vi "iTCread.vi"(0 "VISA resource name":refnum<visa-resource-name>, 1 "iTCreadCtrl":T1, 3 "error in (no error)":errorcluster) -> (7 "VISA resource name out":refnum<visa-resource-name>, 8 "number":dbl, 9 "read buffer":string, 10 "error out":errorcluster)   [LabVIEW 2017]
uses:
  controls/iTCreadCtrl.ctl
  <vilib>/regexp/Match Regular Expression.xnode
panel:
  out "read buffer 2":string
  out "after match":string
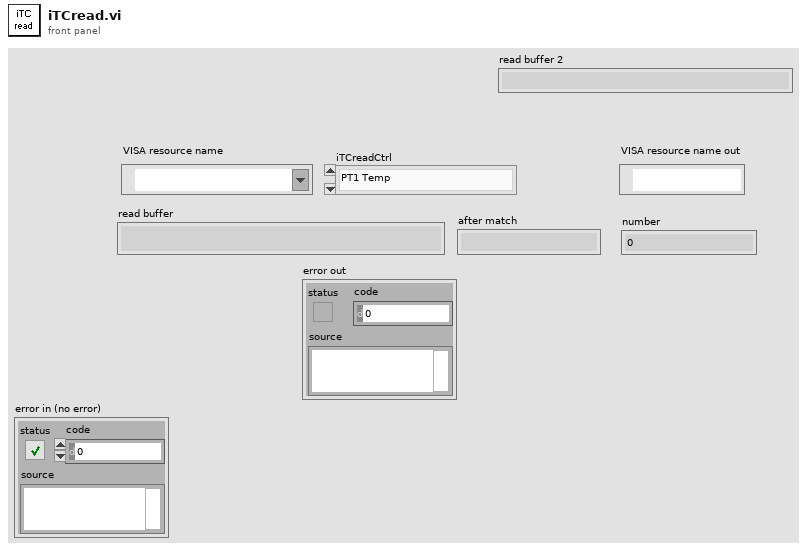
[diagram p1: front panel]
types:
  T1 = typedef "iTCreadCtrl.ctl" = enum16{"PT1 Temp", "PT2 Temp", "Sample Temp", "VTI Temp", "Needle Valve", "VTI Heater Power", "Sample Heater Power", "VTI Pressure"}
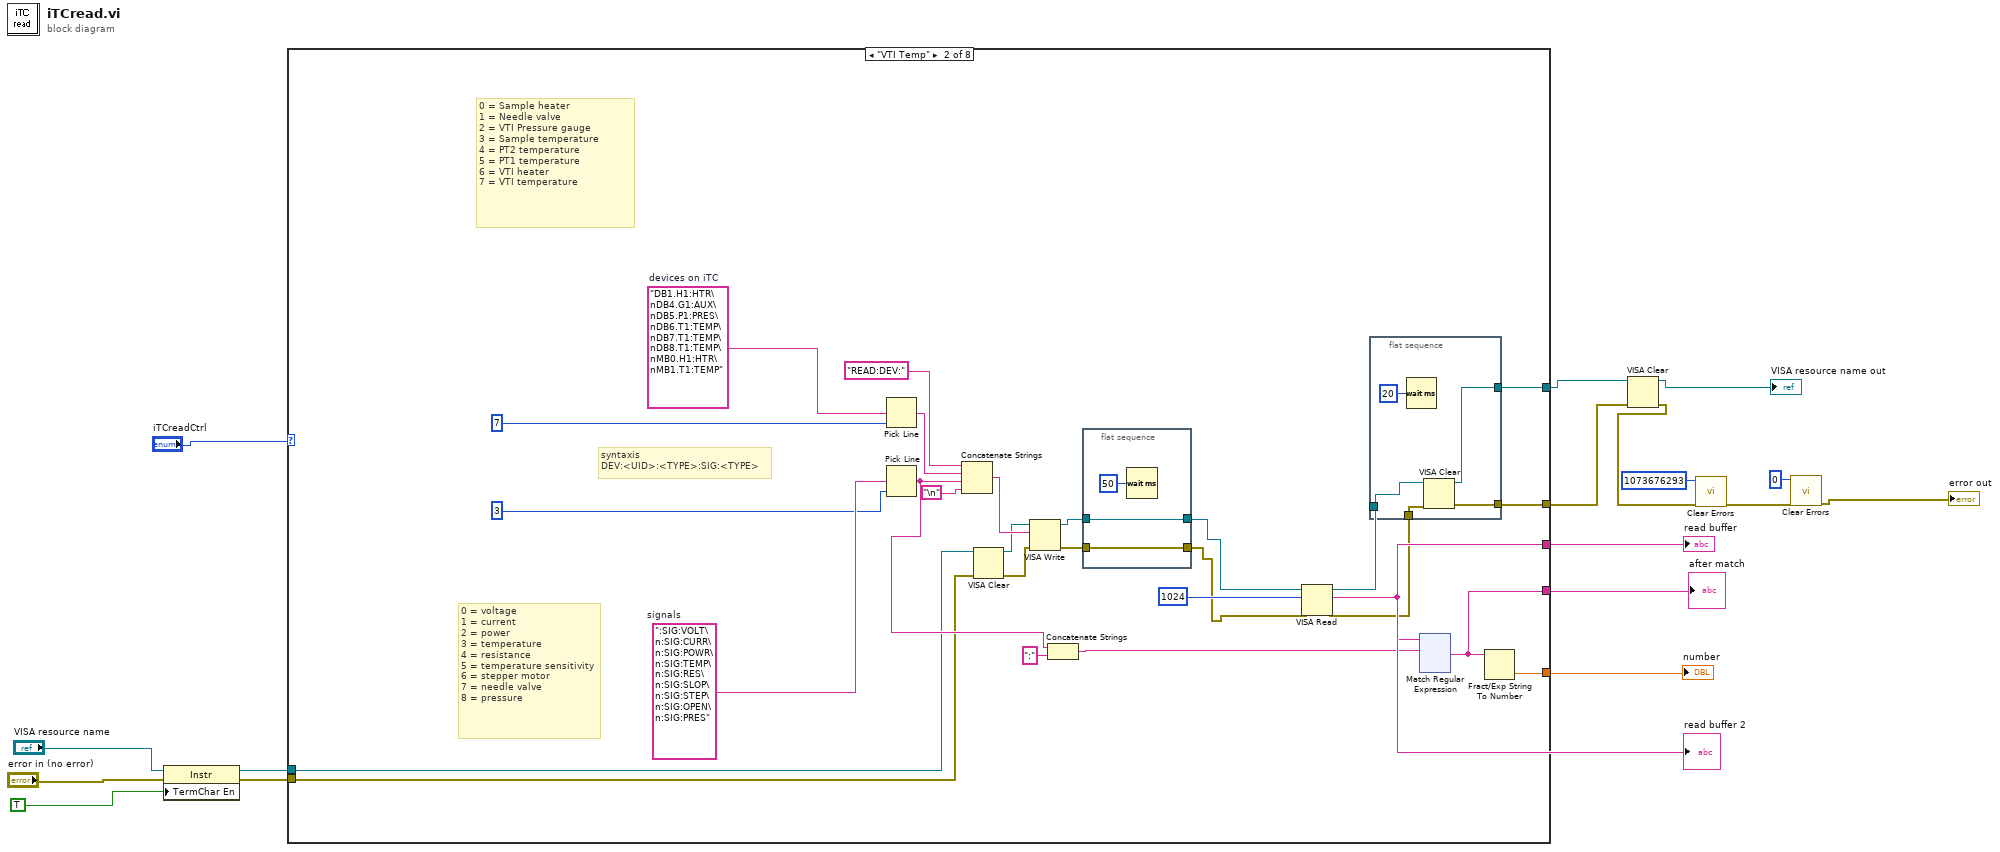
[diagram p0: block diagram]
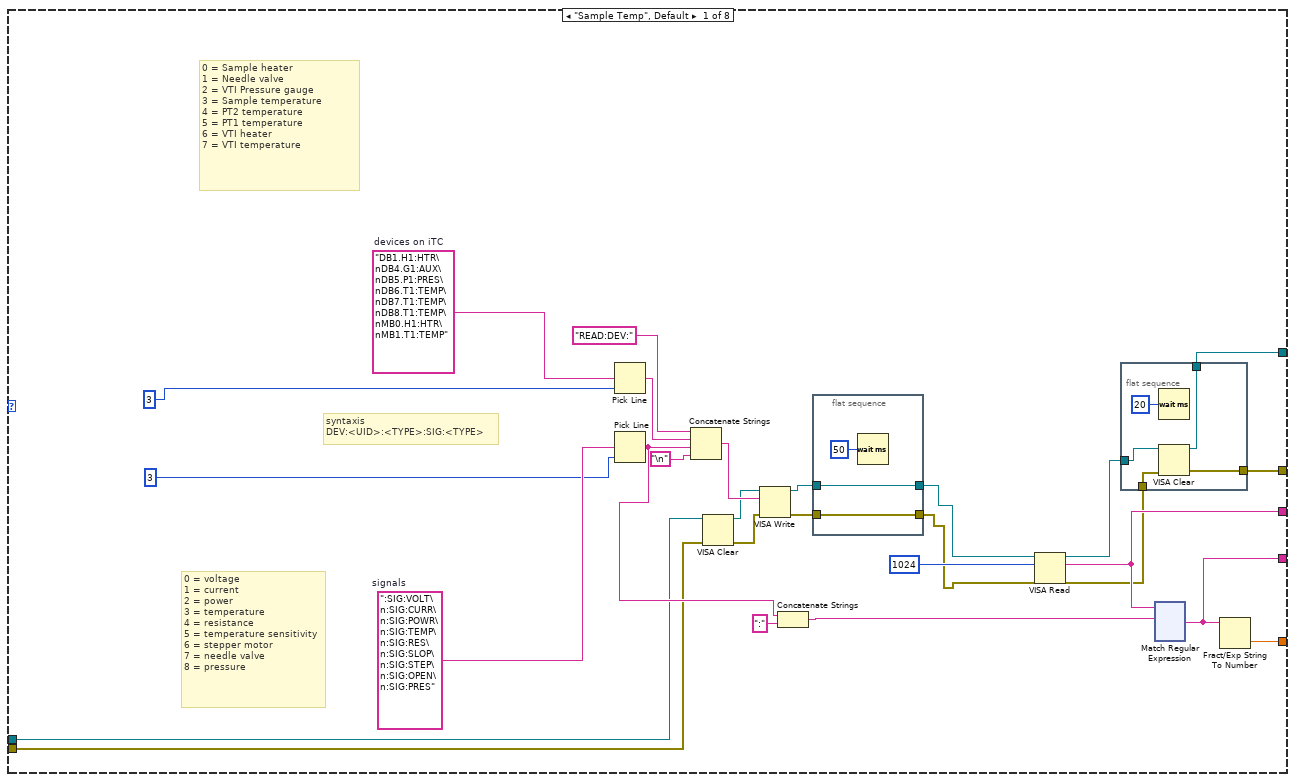
[diagram p2: hidden frame]
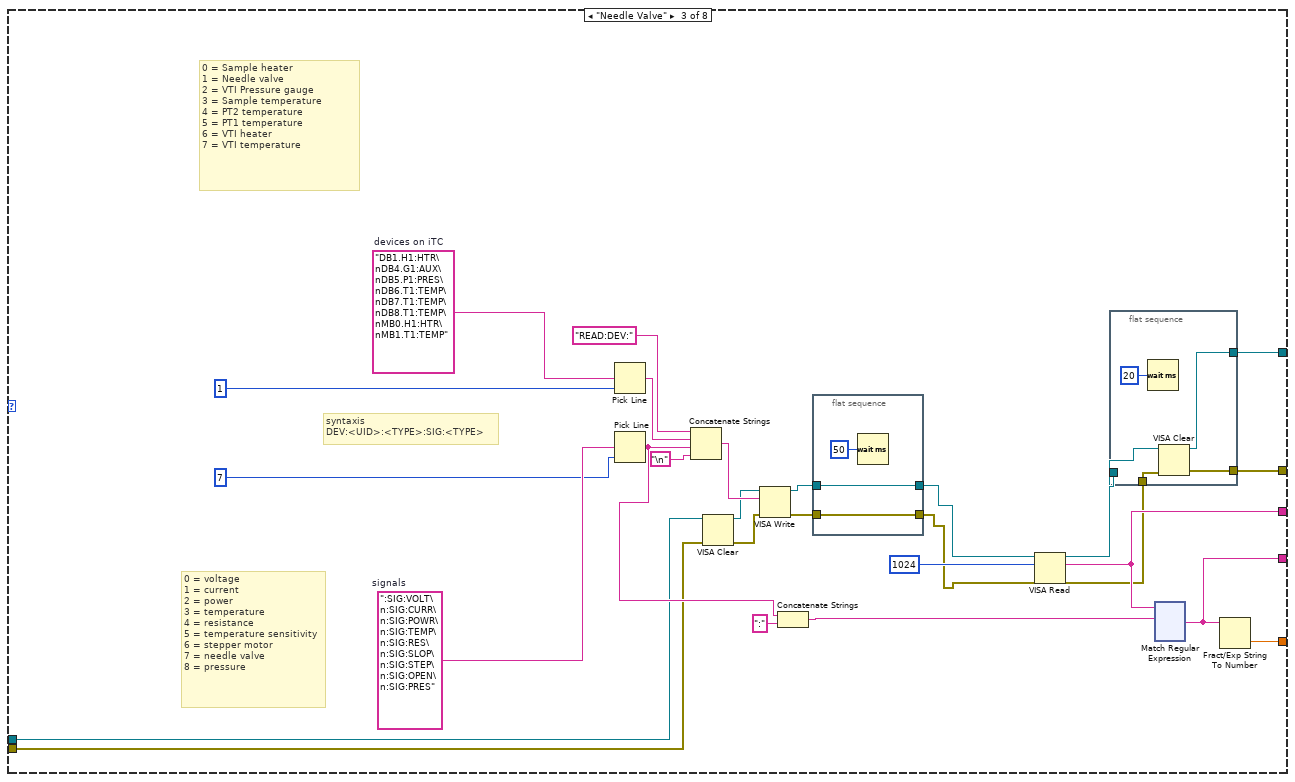
[diagram p3: hidden frame]
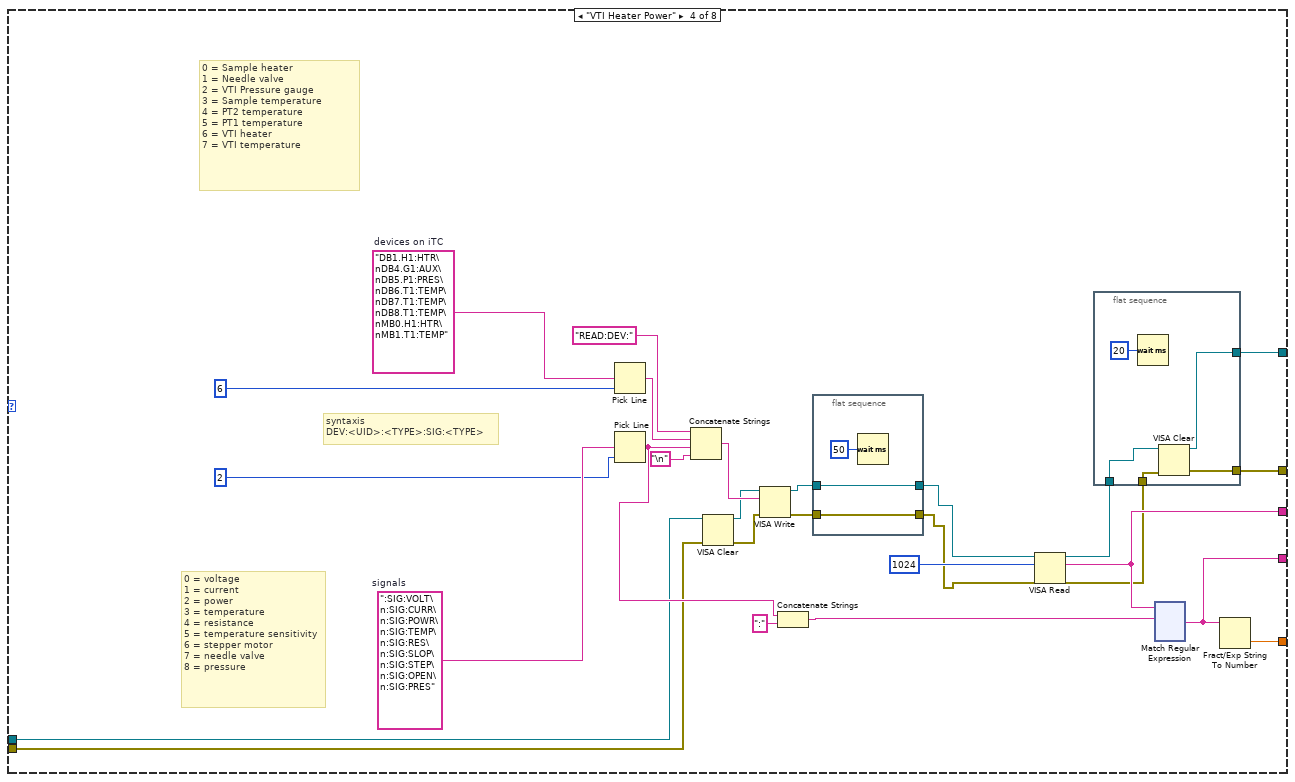
[diagram p4: hidden frame]
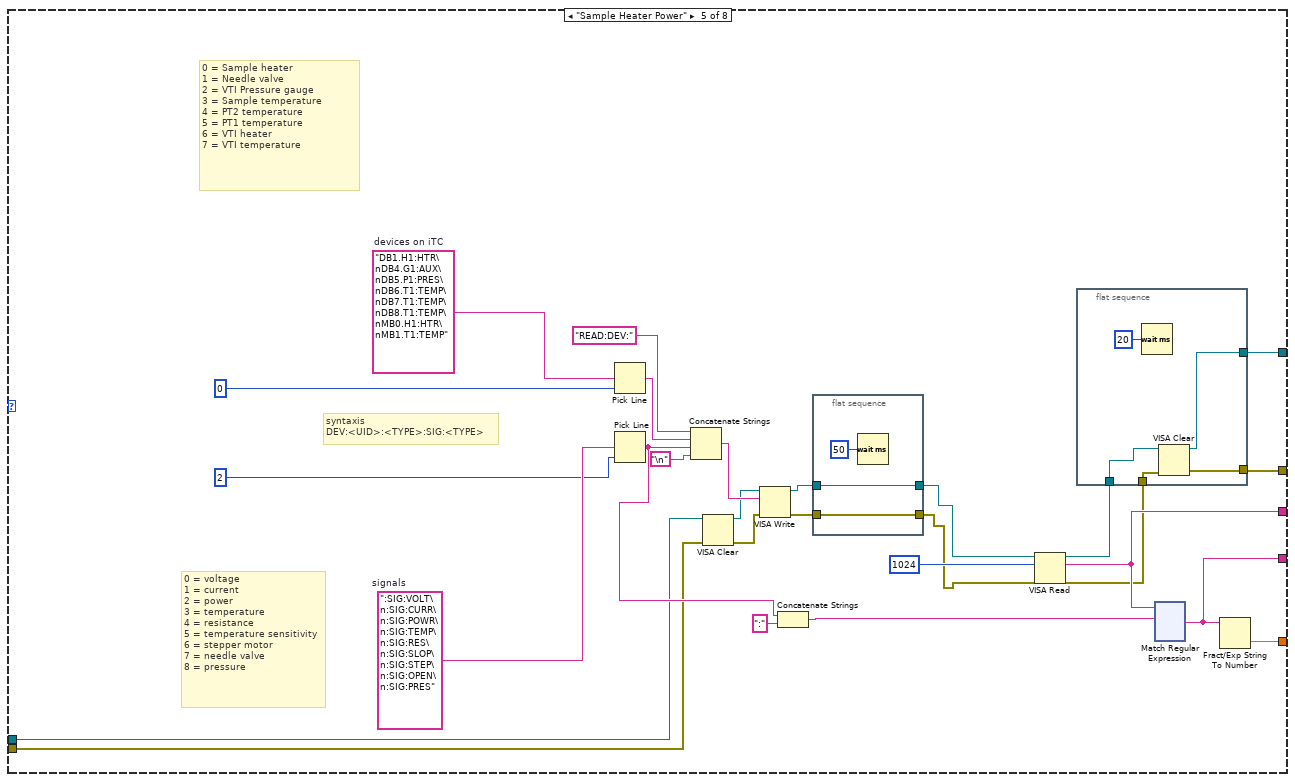
[diagram p5: hidden frame]
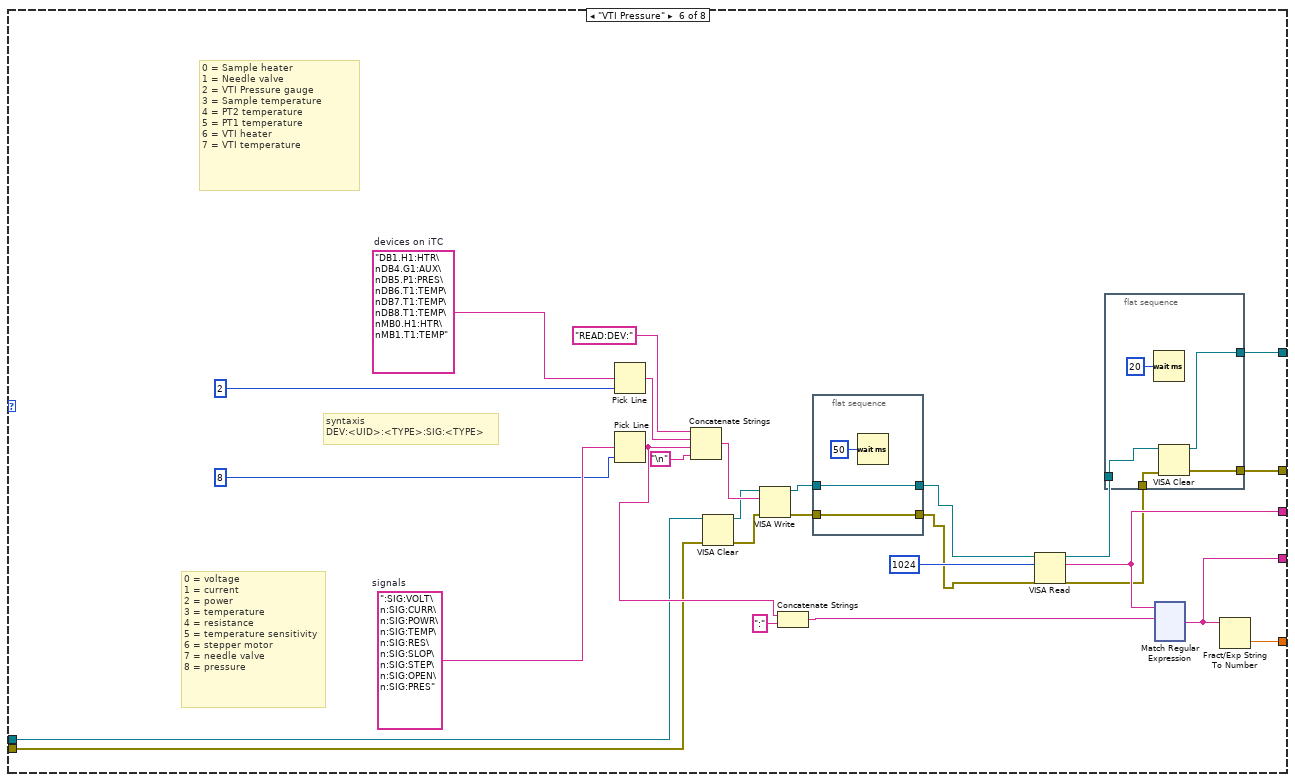
[diagram p6: hidden frame]
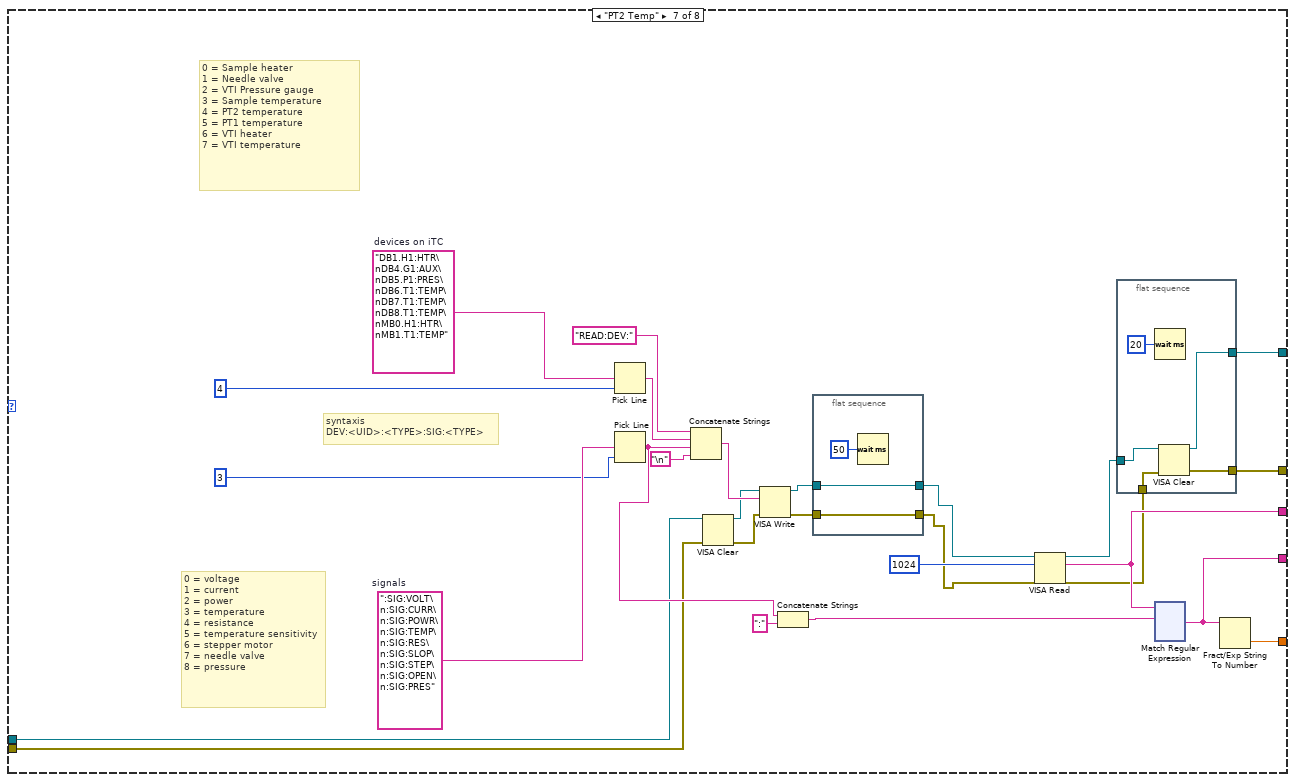
[diagram p7: hidden frame]
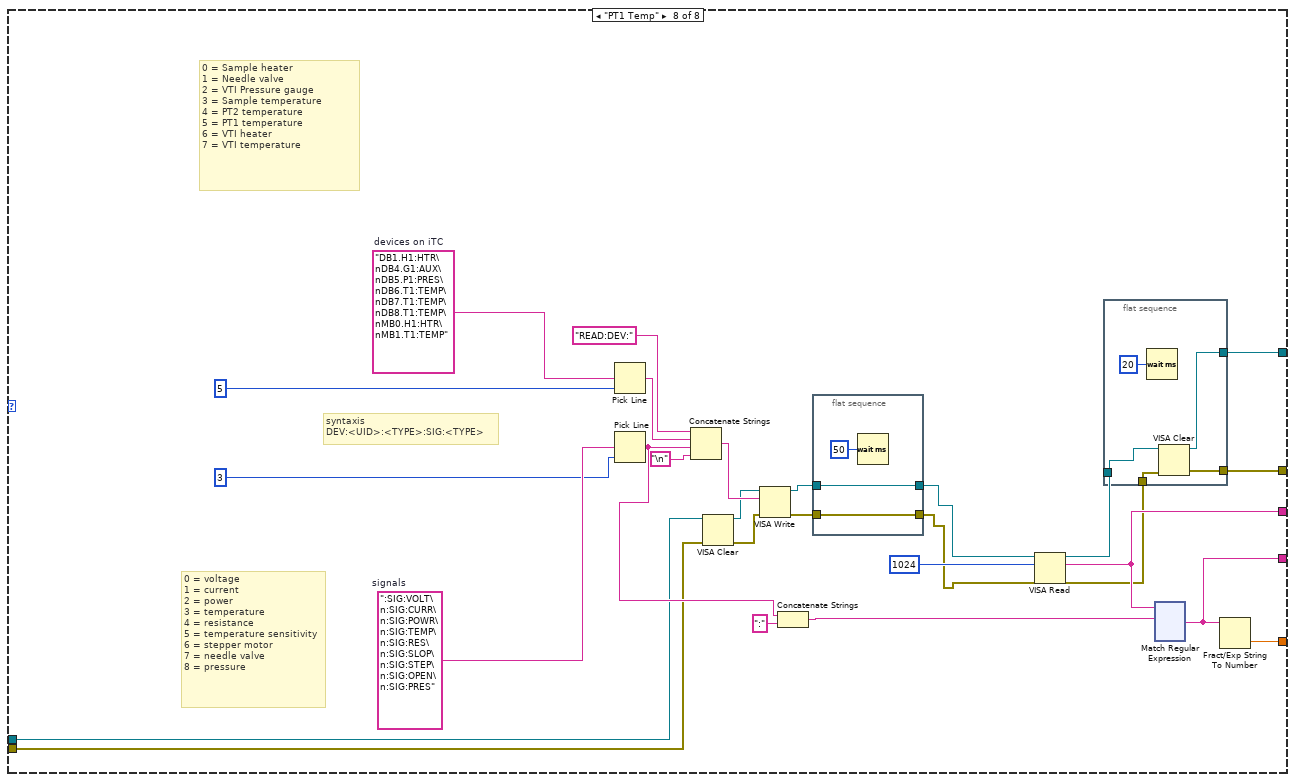
[diagram p8: hidden frame]
diagram:
  n1 = property class="Instr"(reference="VISA resource name", error in="error in (no error)", "TermChar En"=TRUE ("Message Based Settings:Termination Character Enable")) -> (reference out=w11:refnum<visa-resource-name>, error out=w12:errorcluster)
  n2 = case shown="\"VTI Temp\"" "iTCreadCtrl" {
    tunnel: [w44 w190 w336 w482 w628 w774 w920 w1066] -> w17
    tunnel: [w43 w189 w335 w481 w627 w773 w919 w1065] -> w16
    tunnel: [w42 w188 w334 w480 w626 w772 w918 w1064] -> w15
    tunnel: [w41 w187 w333 w479 w625 w771 w917 w1063] -> w2
    tunnel: [w40 w186 w332 w478 w624 w770 w916 w1062] -> w4
    tunnel: w12 -> [w23 w169 w315 w461 w607 w753 w899 w1045]
    tunnel: w11 -> [w22 w168 w314 w460 w606 w752 w898 w1044]
    frame "Sample Temp", Default {
      w36 = ":SIG:VOLT\n:SIG:CURR\n:SIG:POWR\n:SIG:TEMP\n:SIG:RES\n:SIG:SLOP\n:SIG:STEP\n:SIG:OPEN\n:SIG:PRES"  # signals
      w39 = "DB1.H1:HTR\nDB4.G1:AUX\nDB5.P1:PRES\nDB6.T1:TEMP\nDB7.T1:TEMP\nDB8.T1:TEMP\nMB0.H1:HTR\nMB1.T1:TEMP"  # devices on iTC
      # "0 = Sample heater\n1 = Needle valve\n2 = VTI Pressure gauge\n3 = Sample temperature\n4 = PT2 temperature\n5 = PT1 temperature\n6 = VTI heater\n7 = VTI temperature"
      # "0 = voltage\n1 = current\n2 = power\n3 = temperature\n4 = resistance\n5 = temperature sensitivity\n6 = stepper motor\n7 = needle valve\n8 = pressure"
      # "syntaxis\nDEV:<UID>:<TYPE>:SIG:<TYPE>"
      n3 = Pick Line(multi-line string=w39, line index=3) -> (output string=w37:string)  [unwired: 1 in]
      n4 = Pick Line(multi-line string=w36, line index=3) -> (output string=w33:string)  [unwired: 1 in]
      n5 = Concatenate Strings("READ:DEV:" ("write buffer"), w37, w33, "\n") -> (w35:string)
      n6 = VISA Clear(VISA resource name=w22, error in (no error)=w23) -> (VISA resource name out=w26:refnum<visa-resource-name>, error out=w27:errorcluster)
      n7 = VISA Write(VISA resource name=w26, write buffer=w35, error in (no error)=w27) -> (VISA resource name out=w21:refnum<visa-resource-name>, error out=w20:errorcluster)  [unwired: 1 out]
      n8 = Concatenate Strings(w33, ":" ("string")) -> (w32:string)
      n9 = flat-sequence {
        tunnel: w21 -> [w52]
        tunnel: w20 -> [w51]
        tunnel: [w52] -> w19
        tunnel: [w51] -> w18
        frame #0 {
          n10 = Wait (ms)(milliseconds to wait=u32 50) -> ()  [unwired: 1 out]
        }
      }
      n11 = VISA Read(VISA resource name=w19, byte count=u32 1024, error in (no error)=w18) -> (VISA resource name out=w25:refnum<visa-resource-name>, read buffer=w42:string, error out=w28:errorcluster)  [unwired: 1 out]
      n12 = flat-sequence {
        tunnel: [w49] -> w41
        tunnel: [w48] -> w40
        tunnel: w28 -> [w47]
        tunnel: w25 -> [w46]
        frame #0 {
          n13 = Wait (ms)(milliseconds to wait=u32 20) -> ()  [unwired: 1 out]
          n14 = VISA Clear(VISA resource name=w46, error in (no error)=w47) -> (VISA resource name out=w48:refnum<visa-resource-name>, error out=w49:errorcluster)
        }
      }
      n15 = xnode "Match Regular Expression"("input string"=w42, "regular expression"=w32) -> ("after match"=w44:string)  [unwired: 4 in, 4 out]
      n16 = Fract/Exp String To Number(string=w44) -> (number=w43:dbl)  [unwired: 3 in, 1 out]
    }
    frame "VTI Temp" {
      w182 = ":SIG:VOLT\n:SIG:CURR\n:SIG:POWR\n:SIG:TEMP\n:SIG:RES\n:SIG:SLOP\n:SIG:STEP\n:SIG:OPEN\n:SIG:PRES"  # signals
      w185 = "DB1.H1:HTR\nDB4.G1:AUX\nDB5.P1:PRES\nDB6.T1:TEMP\nDB7.T1:TEMP\nDB8.T1:TEMP\nMB0.H1:HTR\nMB1.T1:TEMP"  # devices on iTC
      # "0 = Sample heater\n1 = Needle valve\n2 = VTI Pressure gauge\n3 = Sample temperature\n4 = PT2 temperature\n5 = PT1 temperature\n6 = VTI heater\n7 = VTI temperature"
      # "0 = voltage\n1 = current\n2 = power\n3 = temperature\n4 = resistance\n5 = temperature sensitivity\n6 = stepper motor\n7 = needle valve\n8 = pressure"
      # "syntaxis\nDEV:<UID>:<TYPE>:SIG:<TYPE>"
      n17 = Pick Line(multi-line string=w185, line index=7) -> (output string=w183:string)  [unwired: 1 in]
      n18 = Pick Line(multi-line string=w182, line index=3) -> (output string=w179:string)  [unwired: 1 in]
      n19 = Concatenate Strings("READ:DEV:" ("write buffer"), w183, w179, "\n") -> (w181:string)
      n20 = VISA Clear(VISA resource name=w168, error in (no error)=w169) -> (VISA resource name out=w172:refnum<visa-resource-name>, error out=w173:errorcluster)
      n21 = VISA Write(VISA resource name=w172, write buffer=w181, error in (no error)=w173) -> (VISA resource name out=w167:refnum<visa-resource-name>, error out=w166:errorcluster)  [unwired: 1 out]
      n22 = Concatenate Strings(w179, ":" ("string")) -> (w178:string)
      n23 = flat-sequence {
        tunnel: w167 -> [w198]
        tunnel: w166 -> [w197]
        tunnel: [w198] -> w165
        tunnel: [w197] -> w164
        frame #0 {
          n24 = Wait (ms)(milliseconds to wait=u32 50) -> ()  [unwired: 1 out]
        }
      }
      n25 = VISA Read(VISA resource name=w165, byte count=u32 1024, error in (no error)=w164) -> (VISA resource name out=w171:refnum<visa-resource-name>, read buffer=w188:string, error out=w174:errorcluster)  [unwired: 1 out]
      n26 = flat-sequence {
        tunnel: [w195] -> w187
        tunnel: [w194] -> w186
        tunnel: w174 -> [w193]
        tunnel: w171 -> [w192]
        frame #0 {
          n27 = Wait (ms)(milliseconds to wait=u32 20) -> ()  [unwired: 1 out]
          n28 = VISA Clear(VISA resource name=w192, error in (no error)=w193) -> (VISA resource name out=w194:refnum<visa-resource-name>, error out=w195:errorcluster)
        }
      }
      n29 = xnode "Match Regular Expression"("input string"=w188, "regular expression"=w178) -> ("after match"=w190:string)  [unwired: 4 in, 4 out]
      n30 = Fract/Exp String To Number(string=w190) -> (number=w189:dbl)  [unwired: 3 in, 1 out]
    }
    frame "Needle Valve" {
      w328 = ":SIG:VOLT\n:SIG:CURR\n:SIG:POWR\n:SIG:TEMP\n:SIG:RES\n:SIG:SLOP\n:SIG:STEP\n:SIG:OPEN\n:SIG:PRES"  # signals
      w331 = "DB1.H1:HTR\nDB4.G1:AUX\nDB5.P1:PRES\nDB6.T1:TEMP\nDB7.T1:TEMP\nDB8.T1:TEMP\nMB0.H1:HTR\nMB1.T1:TEMP"  # devices on iTC
      # "0 = Sample heater\n1 = Needle valve\n2 = VTI Pressure gauge\n3 = Sample temperature\n4 = PT2 temperature\n5 = PT1 temperature\n6 = VTI heater\n7 = VTI temperature"
      # "0 = voltage\n1 = current\n2 = power\n3 = temperature\n4 = resistance\n5 = temperature sensitivity\n6 = stepper motor\n7 = needle valve\n8 = pressure"
      # "syntaxis\nDEV:<UID>:<TYPE>:SIG:<TYPE>"
      n31 = Pick Line(multi-line string=w331, line index=1) -> (output string=w329:string)  [unwired: 1 in]
      n32 = Pick Line(multi-line string=w328, line index=7) -> (output string=w325:string)  [unwired: 1 in]
      n33 = Concatenate Strings("READ:DEV:" ("write buffer"), w329, w325, "\n") -> (w327:string)
      n34 = VISA Clear(VISA resource name=w314, error in (no error)=w315) -> (VISA resource name out=w318:refnum<visa-resource-name>, error out=w319:errorcluster)
      n35 = VISA Write(VISA resource name=w318, write buffer=w327, error in (no error)=w319) -> (VISA resource name out=w313:refnum<visa-resource-name>, error out=w312:errorcluster)  [unwired: 1 out]
      n36 = Concatenate Strings(w325, ":" ("string")) -> (w324:string)
      n37 = flat-sequence {
        tunnel: w313 -> [w344]
        tunnel: w312 -> [w343]
        tunnel: [w344] -> w311
        tunnel: [w343] -> w310
        frame #0 {
          n38 = Wait (ms)(milliseconds to wait=u32 50) -> ()  [unwired: 1 out]
        }
      }
      n39 = VISA Read(VISA resource name=w311, byte count=u32 1024, error in (no error)=w310) -> (VISA resource name out=w317:refnum<visa-resource-name>, read buffer=w334:string, error out=w320:errorcluster)  [unwired: 1 out]
      n40 = flat-sequence {
        tunnel: [w341] -> w333
        tunnel: [w340] -> w332
        tunnel: w320 -> [w339]
        tunnel: w317 -> [w338]
        frame #0 {
          n41 = Wait (ms)(milliseconds to wait=u32 20) -> ()  [unwired: 1 out]
          n42 = VISA Clear(VISA resource name=w338, error in (no error)=w339) -> (VISA resource name out=w340:refnum<visa-resource-name>, error out=w341:errorcluster)
        }
      }
      n43 = xnode "Match Regular Expression"("input string"=w334, "regular expression"=w324) -> ("after match"=w336:string)  [unwired: 4 in, 4 out]
      n44 = Fract/Exp String To Number(string=w336) -> (number=w335:dbl)  [unwired: 3 in, 1 out]
    }
    frame "VTI Heater Power" {
      w474 = ":SIG:VOLT\n:SIG:CURR\n:SIG:POWR\n:SIG:TEMP\n:SIG:RES\n:SIG:SLOP\n:SIG:STEP\n:SIG:OPEN\n:SIG:PRES"  # signals
      w477 = "DB1.H1:HTR\nDB4.G1:AUX\nDB5.P1:PRES\nDB6.T1:TEMP\nDB7.T1:TEMP\nDB8.T1:TEMP\nMB0.H1:HTR\nMB1.T1:TEMP"  # devices on iTC
      # "0 = Sample heater\n1 = Needle valve\n2 = VTI Pressure gauge\n3 = Sample temperature\n4 = PT2 temperature\n5 = PT1 temperature\n6 = VTI heater\n7 = VTI temperature"
      # "0 = voltage\n1 = current\n2 = power\n3 = temperature\n4 = resistance\n5 = temperature sensitivity\n6 = stepper motor\n7 = needle valve\n8 = pressure"
      # "syntaxis\nDEV:<UID>:<TYPE>:SIG:<TYPE>"
      n45 = Pick Line(multi-line string=w477, line index=6) -> (output string=w475:string)  [unwired: 1 in]
      n46 = Pick Line(multi-line string=w474, line index=2) -> (output string=w471:string)  [unwired: 1 in]
      n47 = Concatenate Strings("READ:DEV:" ("write buffer"), w475, w471, "\n") -> (w473:string)
      n48 = VISA Clear(VISA resource name=w460, error in (no error)=w461) -> (VISA resource name out=w464:refnum<visa-resource-name>, error out=w465:errorcluster)
      n49 = VISA Write(VISA resource name=w464, write buffer=w473, error in (no error)=w465) -> (VISA resource name out=w459:refnum<visa-resource-name>, error out=w458:errorcluster)  [unwired: 1 out]
      n50 = Concatenate Strings(w471, ":" ("string")) -> (w470:string)
      n51 = flat-sequence {
        tunnel: w459 -> [w490]
        tunnel: w458 -> [w489]
        tunnel: [w490] -> w457
        tunnel: [w489] -> w456
        frame #0 {
          n52 = Wait (ms)(milliseconds to wait=u32 50) -> ()  [unwired: 1 out]
        }
      }
      n53 = VISA Read(VISA resource name=w457, byte count=u32 1024, error in (no error)=w456) -> (VISA resource name out=w463:refnum<visa-resource-name>, read buffer=w480:string, error out=w466:errorcluster)  [unwired: 1 out]
      n54 = flat-sequence {
        tunnel: [w487] -> w479
        tunnel: [w486] -> w478
        tunnel: w466 -> [w485]
        tunnel: w463 -> [w484]
        frame #0 {
          n55 = Wait (ms)(milliseconds to wait=u32 20) -> ()  [unwired: 1 out]
          n56 = VISA Clear(VISA resource name=w484, error in (no error)=w485) -> (VISA resource name out=w486:refnum<visa-resource-name>, error out=w487:errorcluster)
        }
      }
      n57 = xnode "Match Regular Expression"("input string"=w480, "regular expression"=w470) -> ("after match"=w482:string)  [unwired: 4 in, 4 out]
      n58 = Fract/Exp String To Number(string=w482) -> (number=w481:dbl)  [unwired: 3 in, 1 out]
    }
    frame "Sample Heater Power" {
      w620 = ":SIG:VOLT\n:SIG:CURR\n:SIG:POWR\n:SIG:TEMP\n:SIG:RES\n:SIG:SLOP\n:SIG:STEP\n:SIG:OPEN\n:SIG:PRES"  # signals
      w623 = "DB1.H1:HTR\nDB4.G1:AUX\nDB5.P1:PRES\nDB6.T1:TEMP\nDB7.T1:TEMP\nDB8.T1:TEMP\nMB0.H1:HTR\nMB1.T1:TEMP"  # devices on iTC
      # "0 = Sample heater\n1 = Needle valve\n2 = VTI Pressure gauge\n3 = Sample temperature\n4 = PT2 temperature\n5 = PT1 temperature\n6 = VTI heater\n7 = VTI temperature"
      # "0 = voltage\n1 = current\n2 = power\n3 = temperature\n4 = resistance\n5 = temperature sensitivity\n6 = stepper motor\n7 = needle valve\n8 = pressure"
      # "syntaxis\nDEV:<UID>:<TYPE>:SIG:<TYPE>"
      n59 = Pick Line(multi-line string=w623, line index=0) -> (output string=w621:string)  [unwired: 1 in]
      n60 = Pick Line(multi-line string=w620, line index=2) -> (output string=w617:string)  [unwired: 1 in]
      n61 = Concatenate Strings("READ:DEV:" ("write buffer"), w621, w617, "\n") -> (w619:string)
      n62 = VISA Clear(VISA resource name=w606, error in (no error)=w607) -> (VISA resource name out=w610:refnum<visa-resource-name>, error out=w611:errorcluster)
      n63 = VISA Write(VISA resource name=w610, write buffer=w619, error in (no error)=w611) -> (VISA resource name out=w605:refnum<visa-resource-name>, error out=w604:errorcluster)  [unwired: 1 out]
      n64 = Concatenate Strings(w617, ":" ("string")) -> (w616:string)
      n65 = flat-sequence {
        tunnel: w605 -> [w636]
        tunnel: w604 -> [w635]
        tunnel: [w636] -> w603
        tunnel: [w635] -> w602
        frame #0 {
          n66 = Wait (ms)(milliseconds to wait=u32 50) -> ()  [unwired: 1 out]
        }
      }
      n67 = VISA Read(VISA resource name=w603, byte count=u32 1024, error in (no error)=w602) -> (VISA resource name out=w609:refnum<visa-resource-name>, read buffer=w626:string, error out=w612:errorcluster)  [unwired: 1 out]
      n68 = flat-sequence {
        tunnel: [w633] -> w625
        tunnel: [w632] -> w624
        tunnel: w612 -> [w631]
        tunnel: w609 -> [w630]
        frame #0 {
          n69 = Wait (ms)(milliseconds to wait=u32 20) -> ()  [unwired: 1 out]
          n70 = VISA Clear(VISA resource name=w630, error in (no error)=w631) -> (VISA resource name out=w632:refnum<visa-resource-name>, error out=w633:errorcluster)
        }
      }
      n71 = xnode "Match Regular Expression"("input string"=w626, "regular expression"=w616) -> ("after match"=w628:string)  [unwired: 4 in, 4 out]
      n72 = Fract/Exp String To Number(string=w628) -> (number=w627:dbl)  [unwired: 3 in, 1 out]
    }
    frame "VTI Pressure" {
      w766 = ":SIG:VOLT\n:SIG:CURR\n:SIG:POWR\n:SIG:TEMP\n:SIG:RES\n:SIG:SLOP\n:SIG:STEP\n:SIG:OPEN\n:SIG:PRES"  # signals
      w769 = "DB1.H1:HTR\nDB4.G1:AUX\nDB5.P1:PRES\nDB6.T1:TEMP\nDB7.T1:TEMP\nDB8.T1:TEMP\nMB0.H1:HTR\nMB1.T1:TEMP"  # devices on iTC
      # "0 = Sample heater\n1 = Needle valve\n2 = VTI Pressure gauge\n3 = Sample temperature\n4 = PT2 temperature\n5 = PT1 temperature\n6 = VTI heater\n7 = VTI temperature"
      # "0 = voltage\n1 = current\n2 = power\n3 = temperature\n4 = resistance\n5 = temperature sensitivity\n6 = stepper motor\n7 = needle valve\n8 = pressure"
      # "syntaxis\nDEV:<UID>:<TYPE>:SIG:<TYPE>"
      n73 = Pick Line(multi-line string=w769, line index=2) -> (output string=w767:string)  [unwired: 1 in]
      n74 = Pick Line(multi-line string=w766, line index=8) -> (output string=w763:string)  [unwired: 1 in]
      n75 = Concatenate Strings("READ:DEV:" ("write buffer"), w767, w763, "\n") -> (w765:string)
      n76 = VISA Clear(VISA resource name=w752, error in (no error)=w753) -> (VISA resource name out=w756:refnum<visa-resource-name>, error out=w757:errorcluster)
      n77 = VISA Write(VISA resource name=w756, write buffer=w765, error in (no error)=w757) -> (VISA resource name out=w751:refnum<visa-resource-name>, error out=w750:errorcluster)  [unwired: 1 out]
      n78 = Concatenate Strings(w763, ":" ("string")) -> (w762:string)
      n79 = flat-sequence {
        tunnel: w751 -> [w782]
        tunnel: w750 -> [w781]
        tunnel: [w782] -> w749
        tunnel: [w781] -> w748
        frame #0 {
          n80 = Wait (ms)(milliseconds to wait=u32 50) -> ()  [unwired: 1 out]
        }
      }
      n81 = VISA Read(VISA resource name=w749, byte count=u32 1024, error in (no error)=w748) -> (VISA resource name out=w755:refnum<visa-resource-name>, read buffer=w772:string, error out=w758:errorcluster)  [unwired: 1 out]
      n82 = flat-sequence {
        tunnel: [w779] -> w771
        tunnel: [w778] -> w770
        tunnel: w758 -> [w777]
        tunnel: w755 -> [w776]
        frame #0 {
          n83 = Wait (ms)(milliseconds to wait=u32 20) -> ()  [unwired: 1 out]
          n84 = VISA Clear(VISA resource name=w776, error in (no error)=w777) -> (VISA resource name out=w778:refnum<visa-resource-name>, error out=w779:errorcluster)
        }
      }
      n85 = xnode "Match Regular Expression"("input string"=w772, "regular expression"=w762) -> ("after match"=w774:string)  [unwired: 4 in, 4 out]
      n86 = Fract/Exp String To Number(string=w774) -> (number=w773:dbl)  [unwired: 3 in, 1 out]
    }
    frame "PT2 Temp" {
      w912 = ":SIG:VOLT\n:SIG:CURR\n:SIG:POWR\n:SIG:TEMP\n:SIG:RES\n:SIG:SLOP\n:SIG:STEP\n:SIG:OPEN\n:SIG:PRES"  # signals
      w915 = "DB1.H1:HTR\nDB4.G1:AUX\nDB5.P1:PRES\nDB6.T1:TEMP\nDB7.T1:TEMP\nDB8.T1:TEMP\nMB0.H1:HTR\nMB1.T1:TEMP"  # devices on iTC
      # "0 = Sample heater\n1 = Needle valve\n2 = VTI Pressure gauge\n3 = Sample temperature\n4 = PT2 temperature\n5 = PT1 temperature\n6 = VTI heater\n7 = VTI temperature"
      # "0 = voltage\n1 = current\n2 = power\n3 = temperature\n4 = resistance\n5 = temperature sensitivity\n6 = stepper motor\n7 = needle valve\n8 = pressure"
      # "syntaxis\nDEV:<UID>:<TYPE>:SIG:<TYPE>"
      n87 = Pick Line(multi-line string=w915, line index=4) -> (output string=w913:string)  [unwired: 1 in]
      n88 = Pick Line(multi-line string=w912, line index=3) -> (output string=w909:string)  [unwired: 1 in]
      n89 = Concatenate Strings("READ:DEV:" ("write buffer"), w913, w909, "\n") -> (w911:string)
      n90 = VISA Clear(VISA resource name=w898, error in (no error)=w899) -> (VISA resource name out=w902:refnum<visa-resource-name>, error out=w903:errorcluster)
      n91 = VISA Write(VISA resource name=w902, write buffer=w911, error in (no error)=w903) -> (VISA resource name out=w897:refnum<visa-resource-name>, error out=w896:errorcluster)  [unwired: 1 out]
      n92 = Concatenate Strings(w909, ":" ("string")) -> (w908:string)
      n93 = flat-sequence {
        tunnel: w897 -> [w928]
        tunnel: w896 -> [w927]
        tunnel: [w928] -> w895
        tunnel: [w927] -> w894
        frame #0 {
          n94 = Wait (ms)(milliseconds to wait=u32 50) -> ()  [unwired: 1 out]
        }
      }
      n95 = VISA Read(VISA resource name=w895, byte count=u32 1024, error in (no error)=w894) -> (VISA resource name out=w901:refnum<visa-resource-name>, read buffer=w918:string, error out=w904:errorcluster)  [unwired: 1 out]
      n96 = flat-sequence {
        tunnel: [w925] -> w917
        tunnel: [w924] -> w916
        tunnel: w904 -> [w923]
        tunnel: w901 -> [w922]
        frame #0 {
          n97 = Wait (ms)(milliseconds to wait=u32 20) -> ()  [unwired: 1 out]
          n98 = VISA Clear(VISA resource name=w922, error in (no error)=w923) -> (VISA resource name out=w924:refnum<visa-resource-name>, error out=w925:errorcluster)
        }
      }
      n99 = xnode "Match Regular Expression"("input string"=w918, "regular expression"=w908) -> ("after match"=w920:string)  [unwired: 4 in, 4 out]
      n100 = Fract/Exp String To Number(string=w920) -> (number=w919:dbl)  [unwired: 3 in, 1 out]
    }
    frame "PT1 Temp" {
      w1058 = ":SIG:VOLT\n:SIG:CURR\n:SIG:POWR\n:SIG:TEMP\n:SIG:RES\n:SIG:SLOP\n:SIG:STEP\n:SIG:OPEN\n:SIG:PRES"  # signals
      w1061 = "DB1.H1:HTR\nDB4.G1:AUX\nDB5.P1:PRES\nDB6.T1:TEMP\nDB7.T1:TEMP\nDB8.T1:TEMP\nMB0.H1:HTR\nMB1.T1:TEMP"  # devices on iTC
      # "0 = Sample heater\n1 = Needle valve\n2 = VTI Pressure gauge\n3 = Sample temperature\n4 = PT2 temperature\n5 = PT1 temperature\n6 = VTI heater\n7 = VTI temperature"
      # "0 = voltage\n1 = current\n2 = power\n3 = temperature\n4 = resistance\n5 = temperature sensitivity\n6 = stepper motor\n7 = needle valve\n8 = pressure"
      # "syntaxis\nDEV:<UID>:<TYPE>:SIG:<TYPE>"
      n101 = Pick Line(multi-line string=w1061, line index=5) -> (output string=w1059:string)  [unwired: 1 in]
      n102 = Pick Line(multi-line string=w1058, line index=3) -> (output string=w1055:string)  [unwired: 1 in]
      n103 = Concatenate Strings("READ:DEV:" ("write buffer"), w1059, w1055, "\n") -> (w1057:string)
      n104 = VISA Clear(VISA resource name=w1044, error in (no error)=w1045) -> (VISA resource name out=w1048:refnum<visa-resource-name>, error out=w1049:errorcluster)
      n105 = VISA Write(VISA resource name=w1048, write buffer=w1057, error in (no error)=w1049) -> (VISA resource name out=w1043:refnum<visa-resource-name>, error out=w1042:errorcluster)  [unwired: 1 out]
      n106 = Concatenate Strings(w1055, ":" ("string")) -> (w1054:string)
      n107 = flat-sequence {
        tunnel: w1043 -> [w1074]
        tunnel: w1042 -> [w1073]
        tunnel: [w1074] -> w1041
        tunnel: [w1073] -> w1040
        frame #0 {
          n108 = Wait (ms)(milliseconds to wait=u32 50) -> ()  [unwired: 1 out]
        }
      }
      n109 = VISA Read(VISA resource name=w1041, byte count=u32 1024, error in (no error)=w1040) -> (VISA resource name out=w1047:refnum<visa-resource-name>, read buffer=w1064:string, error out=w1050:errorcluster)  [unwired: 1 out]
      n110 = flat-sequence {
        tunnel: [w1071] -> w1063
        tunnel: [w1070] -> w1062
        tunnel: w1050 -> [w1069]
        tunnel: w1047 -> [w1068]
        frame #0 {
          n111 = Wait (ms)(milliseconds to wait=u32 20) -> ()  [unwired: 1 out]
          n112 = VISA Clear(VISA resource name=w1068, error in (no error)=w1069) -> (VISA resource name out=w1070:refnum<visa-resource-name>, error out=w1071:errorcluster)
        }
      }
      n113 = xnode "Match Regular Expression"("input string"=w1064, "regular expression"=w1054) -> ("after match"=w1066:string)  [unwired: 4 in, 4 out]
      n114 = Fract/Exp String To Number(string=w1066) -> (number=w1065:dbl)  [unwired: 3 in, 1 out]
    }
  }
  "read buffer" <- w15
  "after match" <- w17
  "number" <- w16
  "read buffer 2" <- w15
  n115 = VISA Clear(VISA resource name=w4, error in (no error)=w2) -> (VISA resource name out=→"VISA resource name out":refnum<visa-resource-name>, error out=w1:errorcluster)
  n116 = call <vilib>:"Clear Errors.vi"("error in (no error)"=w1, "specific error code to clear (0: all)"=1073676293) -> ("error out"=w7:errorcluster)  [unwired: 4 in, 1 out]
  n117 = call <vilib>:"Clear Errors.vi"("error in (no error)"=w7, "specific error code to clear (0: all)"=0) -> ("error out"=→"error out":errorcluster)  [unwired: 4 in, 1 out]
